vi "Entmagnetisierung.vi"(5 "minimale Spannung FG":dbl, 7 "Frequenz":dbl, 8 "error in (no error)":errorcluster, 9 "Spannungsabweichung":dbl, 10 "Wartezeit pro Schritt in ms (250ms)":u32=250, 11 "VISA Name FG in":refnum<visa-resource-name>) -> (0 "error out":errorcluster, 3 "Spannung an FG":dbl)   [LabVIEW 2016]
uses:
  <instrlib>/agilent_33xxx_series/Agilent 33XXX Series/Agilent 33XXX Series.lvlib
panel:
  out "VISA Name FG out":refnum<visa-resource-name>
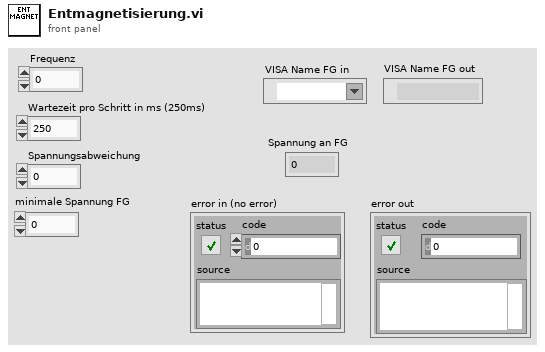
[diagram p1: front panel]
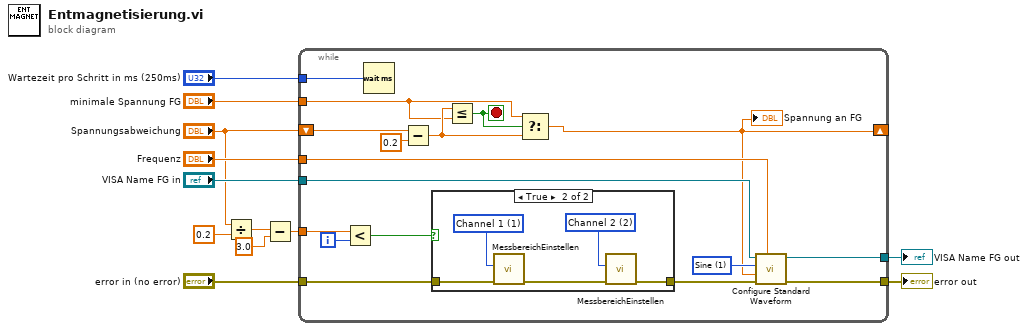
[diagram p0: block diagram]
diagram:
  n1 = Divide(x="Spannungsabweichung", y=0.2) -> (x/y=w4:dbl)
  n2 = Subtract(x=w4, y=3.0) -> (x-y=w1:dbl)
  n3 = while {
    tunnel: "Wartezeit pro Schritt in ms (250ms)" -> [w26]
    tunnel: "error in (no error)" -> [w17]
    tunnel: [w21] -> w10
    tunnel: "VISA Name FG in" -> [w25]
    tunnel: "Frequenz" -> [w24]
    tunnel: [w23] -> w7
    shift-right: [w19] -> _
    shift-left: "Spannungsabweichung" -> [w20]
    tunnel: "minimale Spannung FG" -> [w18]
    tunnel: w1 -> [w13]
    i -> [w14]
    stop <- w22 stop-if-true
    w27 = u16 1 items=["DC", "Sine", "Square", "Triangle", "Ramp", "Pulse", "Noise", "Sinc", "Negative Ramp", "Exponential Rise", "Exponential Fall", "Cardiac"] ("Waveform Function (1: Sine)")
    n4 = Less?(x=w13, y=w14) -> (x < y?=w15:bool)
    n5 = Wait (ms)(milliseconds to wait=w26) -> ()  [unwired: 1 out]
    n6 = Subtract(x=w20, y=0.2) -> (x-y=w28:dbl)
    n7 = case shown="True" w15 {
      tunnel: [w30 w32] -> w16
      tunnel: w17 -> [w30 w31]
      frame False {
      }
      frame True {
        w34 = 2 items=["Channel 1"=1, "Channel 2"=2, "Channel 3"=3, "Channel 4"=4] ("Channel Name (1: Channel 1)")
        w35 = 1 items=["Channel 1"=1, "Channel 2"=2, "Channel 3"=3, "Channel 4"=4] ("Channel Name (1: Channel 1)")
        n8 = call "MessbereichEinstellen.vi"("Error_in"=w31, "Channel Name (1: Channel 1)"=w35) -> ("Error_out"=w33:errorcluster)  [unwired: 8 in, 1 out]
        n9 = call "MessbereichEinstellen.vi"("Error_in"=w33, "Channel Name (1: Channel 1)"=w34) -> ("Error_out"=w32:errorcluster)  [unwired: 8 in, 1 out]
      }
    }
    n10 = Less Or Equal?(x=w28, y=w18) -> (x <= y?=w22:bool)
    n11 = Select(t=w18, s=w22, f=w28) -> (s? t:f=w19:dbl)
    "Spannung an FG" <- w19
    n12 = call <instrlib>:"Configure Standard Waveform.vi"("Frequency (1000 Hz)"=w24, "error in (no error)"=w16, "Amplitude (1)"=w19, "Waveform Function (1: Sine)"=w27, "VISA resource name"=w25) -> ("error out"=w21:errorcluster, "VISA resource name out"=w23:refnum<visa-resource-name>)  [unwired: 5 in]
  }
  "error out" <- w10
  "VISA Name FG out" <- w7
